vi "Display TEDS Data.vi"(3 "TEDS Array":T1(array[cluster])) -> ()   [LabVIEW 2021]
panel:
  out "TEDS Error":string
  out "TEDS Error?":bool
  out "TEDS Data":string[][](table)
  in  "Done":bool
  in  "Select Channel":u16(ring) items=["Channel 0", "Channel 1", "Channel 2", "Channel 3"]
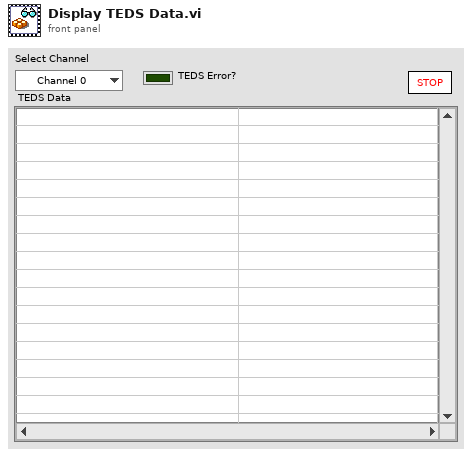
[diagram p1: front panel]
types:
  T1 = cluster{"TEDS Error?":bool, "TEDS Error":string, "TEDS Data":string[][]}[]
  T2 = cluster{"TEDS Error?":bool, "TEDS Error":string, "TEDS Data":string[][]}
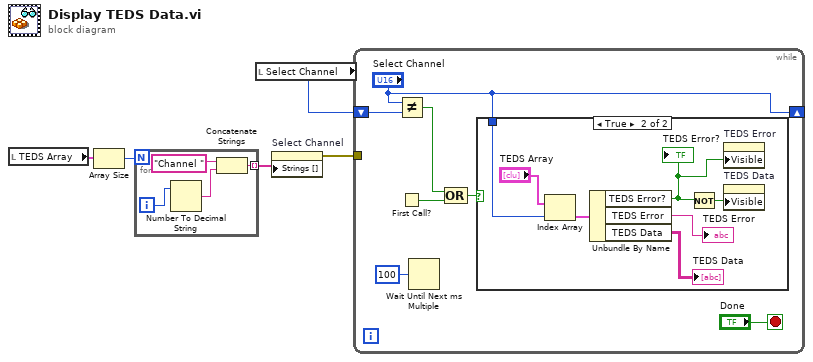
[diagram p0: block diagram]
diagram:
  n1 = local read "TEDS Array"() -> (w4:T1)
  n2 = Array Size(array=w4) -> (size(s)=w3:i32)
  n3 = for {
    N: w3 -> [_]
    tunnel: [w7] -> w2 mode=indexing
    i -> [w6]
    n4 = Number To Decimal String(number=w6) -> (decimal integer string=w8:string)  [unwired: 1 out]
    n5 = Concatenate Strings("Channel ", w8) -> (w7:string)
  }
  n6 = local read "Select Channel"() -> (w5:u16)
  n7 = property on="Select Channel" class="Ring (strict)"("Strings []"=w2) -> (error out=w1:errorcluster)  [unwired: 2 in, 1 out]
  n8 = while {
    shift-right: ["Select Channel"] -> _
    shift-left: w5 -> [w14]
    tunnel: w1 -> [_]
    stop <- "Done" stop-if-true
    n9 = Not Equal?(x="Select Channel", y=w14) -> (x != y?=w13:bool)
    n10 = First Call?() -> (First Call?: T/F=w12:bool)
    n11 = Wait Until Next ms Multiple(millisecond multiple=u32 100) -> ()  [unwired: 1 out]
    n12 = Compound Arithmetic op=OR(w13, w12) -> (w11:bool)
    n13 = case shown="True" w11 {
      tunnel: "Select Channel" -> [_ w23]
      frame False {
      }
      frame True {
        n14 = Index Array(array="TEDS Array", index=w23) -> (element=w21:T2)
        n15 = Unbundle By Name(w21) -> ("TEDS Error?"=w17:bool, "TEDS Error"=→"TEDS Error":string, "TEDS Data"=→"TEDS Data":string[][])
        "TEDS Error?" <- w17
        n16 = Not(x=w17) -> (.not. x?=w18:bool)
        n17 = property on="TEDS Error" class="Str"("Visible"=w17) -> ()  [unwired: 2 in, 2 out]
        n18 = property on="TEDS Data" class="Tbl (strict)"("Visible"=w18) -> ()  [unwired: 2 in, 2 out]
      }
    }
  }
